vi "CBL Open Device.vi"(8 "error in (no error)":errorcluster, 11 "DevIndex":i32) -> (0 "error out":errorcluster, 3 "function return":i32)   [LabVIEW 2012, in "CANBootloader.lvlib"]
doc: "int WINAPI CBL_OpenDevice(int DevIndex);"
uses:
  CANBootloader.lvlib
  Ginkgo_Driver.dll
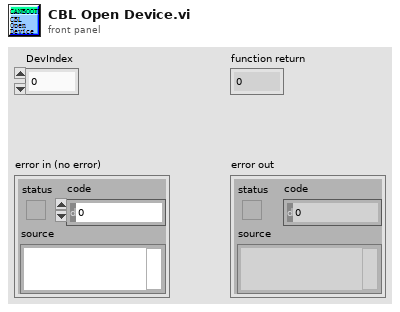
[diagram p1: front panel]
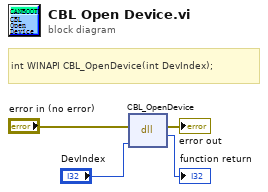
[diagram p0: block diagram]
diagram:
  # "int WINAPI CBL_OpenDevice(int DevIndex);"
  n1 = dll-call lib="E:/Project/vt_ginkgo/truck/Ginkgo Driver/vs2010/Ginkgo_USB-I2C_API_v2.0.3.0/lib/labview_64bit/CANBootloader/Ginkgo_Driver.*" fn="CBL_OpenDevice"(error in="error in (no error)", "DevIndex"="DevIndex") -> (error out=→"error out":errorcluster, →"function return":i32)  [unwired: 3 in, 1 out]
